vi "Duplicate.vi"(8 "error in":errorcluster, 10 "parameters":variant, 11 "FPGA Instrument in":refnum<class "FPGA Instrument.lvclass">) -> (0 "error out":errorcluster, 3 "FPGA Instrument out":refnum<class "FPGA Instrument.lvclass">)   [LabVIEW 2025, in "FPGA.lvlib" / "FPGA Instrument.lvclass"]
doc: "Implements the specific behavior of a node when it is being duplicated\nCan be used to change the name of the new node for example adding Copy to it. \nCopyright 2017 National Instruments Corporation\n\nLicensed under the Apache License, Version 2.0 (the \"License\"); you may not use this file except in compliance with the License. You may obtain a copy of the License at http://www.apache.org/licenses/LICENSE-2.0\nUnless required by applicable law or agreed to in writing, software distributed under the License is distributed on an \"AS IS\" BASIS, WITHOUT WARRANTIES OR CONDITIONS OF ANY KIND, either express or implied. See the License for the specific language governing permissions and limitations under the License."
uses:
  FPGA Instrument.lvclass
  FPGA Instrument.lvclass/FPGA Instrument.ctl
  FPGA configuration/FPGA configuration.lvclass
  C:/Users/Public/Documents/Sandia National Labs/TSS Plugin/Abstract Engine.lvlibp/Instrument configuration/Instrument configuration.lvclass
  Users/Public/Documents/Sandia National Labs/TSS Plugin/Abstract Engine.lvlibp/Instrument configuration/Read Instrument Setting.vi
  Users/Public/Documents/Sandia National Labs/TSS Plugin/Abstract Engine.lvlibp/Instrument configuration/Write Instrument Setting.vi
  Users/Public/Documents/Sandia National Labs/TSS Plugin/Abstract Engine.lvlibp/Abstract Instrument/Abstract Instrument.lvclass
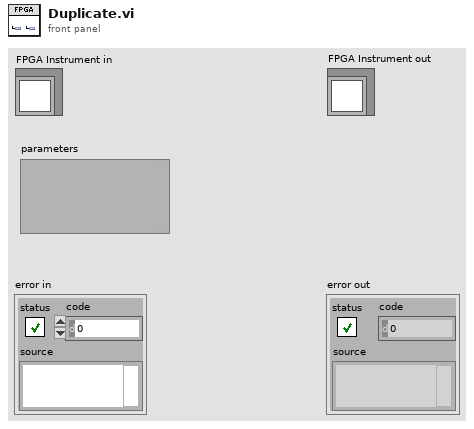
[diagram p1: front panel]
types:
  T1 = typedef "Abstract Engine.lvlibp/Instrument configuration.lvclass/Default Instrument.ctl" = cluster{"Type":string, "Address":string, "SW Alias":string, "Description":string, "Enabled":bool}
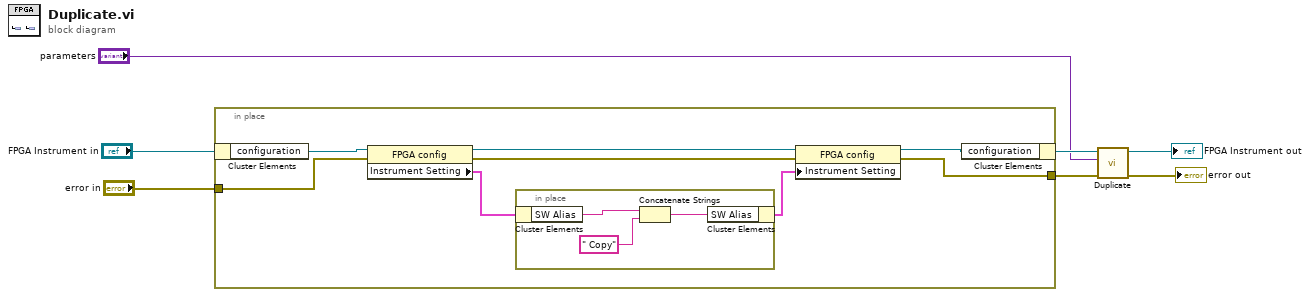
[diagram p0: block diagram]
diagram:
  n1 = in-place {
    in-place-border: "error in" -> [w12]
    in-place-border: [w9] -> w1
    n2 = in-place-cluster #1("FPGA Instrument in") -> ("configuration"=w15:refnum<class "FPGA configuration.lvclass">)
    n3 = property class="FPGA config"(reference=w15, error in=w12) -> (reference out=w13:refnum<class "FPGA configuration.lvclass">, error out=w10:errorcluster, "Instrument Setting"=w11:T1)
    n4 = in-place {
      n5 = in-place-cluster #2(w11) -> ("SW Alias"=w18:string)
      n6 = Concatenate Strings(w18, " Copy") -> (w17:string)
      n7 = in-place-cluster #2("SW Alias"=w17) -> (w8:T1)
    }
    n8 = property class="FPGA config"(reference=w13, error in=w10, "Instrument Setting"=w8) -> (reference out=w14:refnum<class "FPGA configuration.lvclass">, error out=w9:errorcluster)
    n9 = in-place-cluster #1("configuration"=w14) -> (w4:refnum<class "FPGA Instrument.lvclass">)
  }
  n10 = call-parent "Duplicate.vi"("error in"=w1, "parameters"="parameters", "CEF_Serialize node in"=w4) -> ("error out"=→"error out":errorcluster, "CEF_Serialize node out"=→"FPGA Instrument out":refnum<class "FPGA Instrument.lvclass">)  [unwired: 7 in]
